vi "Nod eID handler.vi"(1 "Loop ID":T1, 11 "error in (no error)":errorcluster) -> ()   [LabVIEW 2011]
uses:
  Application Structure/Loop ID.ctl
  Defenitions/LEIN STAT 15 Id system cluster v2 wo lables.ctl
  emi Lib/System 01/0 - General/App/Loop control 2/Private/_emi_ SMLoop start condition.vi
  emi Lib/System 01/0 - General/App/Loop control 2/Private/_emi_ SMLoop Error Check.vi
  emi Lib/Basic/0 - General/Error/emi_Is Error.vi
  emi Lib/System 01/0 - General/App/Loop control 2/Private/_emi_SMLoop Register new.vi
  emi Lib/System 01/0 - General/S&E reporting/emi_Send S&E Error message.vi
  emi Lib/Basic/0 - General/Error/emi_ Is Error state.vi
  emi Lib/System 01/0 - General/emi_Read System ID.vi
  emi Lib/System 01/0 - General/App/Loop control/Private/_emi_GFV Loop Linking.vi
  emi Lib/System 01/0 - General/App/Loop control/Private/_emi_GFV Loop Enable.vi
  emi Lib/System 01/0 - General/App/Loop control 2/Private/_emi_ SMLoop Restart.vi
  emi Lib/System 01/0 - General/App/Private/_emi_GFV App Close.vi
  emi Lib/System 01/0 - General/App/Loop control 2/Private/_emi_ SMLoop Restart Counter.vi
  emi Lib/System 01/0 - General/App/Loop control/Private/_emi_GFV Loop Running.vi
  emi Lib/System 01/0 - General/Private/_emi_GFV System ID.vi
  emi Lib/System 01/0 - General/S&E reporting/Private/_emi_S&E Q Generator.vi
  <vilib>/Utility/error.llb/Clear Errors.vi
  emi Lib/System 01/0 - General/App/Loop control/Private/_emi_GFV stop a loop so it can reset.vi
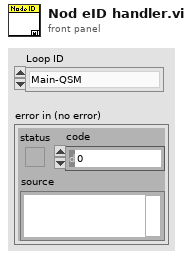
[diagram p1: front panel]
types:
  T1 = typedef "Loop ID.ctl" = enum16{"Main-QSM", "Main-Dialog", "Main-Ind Upd", "Main-Graph Upd", "Main-Debug", "Main-DebugW1", "Main-DebugW2", "Main-SE Handler", "Interface-PCP", "Interface-CANbus", "Interface-Modem", "Var Handling-Beat", "Var Handling-From PCP", "Var Handling-File storage", "Var Handling-From Simulator", "GUI-GrphW Mast", "GUI-GrphW Slav", "SIM-Tool W1", "SIM-Tool W2", "Alm-Sound", "LEIN-motor", "Tool data gatherer Qer", "Tool Data LEIN STAT2 dekoder", "Indicator Value Update", "Tool STAT2 dedicated reader", "Tool ID handler", "Detail View L1", "Detail View L2", "Main display enable view", "Sequence runner", "Voltage setpoint", "Resistance setpoint", "Stroker Wizard L1", "Stroker Wizard L2", "Alarm Handling", "Annotations Tip Strip", "Magna Interface", "Modem Status", "Var Handling - Modem Status", "Power interface detector"}
  T2 = typedef "LEIN STAT 15 Id system cluster v2 wo lables.ctl" = cluster{"LEIN version":u8, "LEIN implementation code":u8, "Serial number":u16, "Project":u16, "HW ID":u8, "FW ID":u8, "HW REV":u8, "FW REV":u8}
  T3 = enum16{"big-endian, network order", "native, host order", "little-endian"}
  T4 = typedef "_emi_ SMLoop sates.ctl" = enum16{"Init", "Standby", "Start", "Normal Operation", "Stop", "Error Handling", "End", "Post"}
  T5 = typedef "LEIN custom reply Q.ctl" = refnum<queue>
  T6 = typedef "LEIN Reply Holder.ctl" = cluster{"Reply msg(cmdif no reply)":T7, "Reply time":timestamp, "Valid reply":bool}
  T7 = typedef "LEIN CMD Cluster.ctl" = cluster{"SID":u8, "ANF":bool, "CMD":T8, "DATA":u8[]}
  T8 = typedef "LEIN CMD List.ctl" = enum8{"ACTI", "TASK", "RES0", "STAT", "RES1", "RES2", "RES3", "USER"}
  T9 = typedef "List of tools.ctl" = enum16{"Stroker", "Driller", "Tractor"}
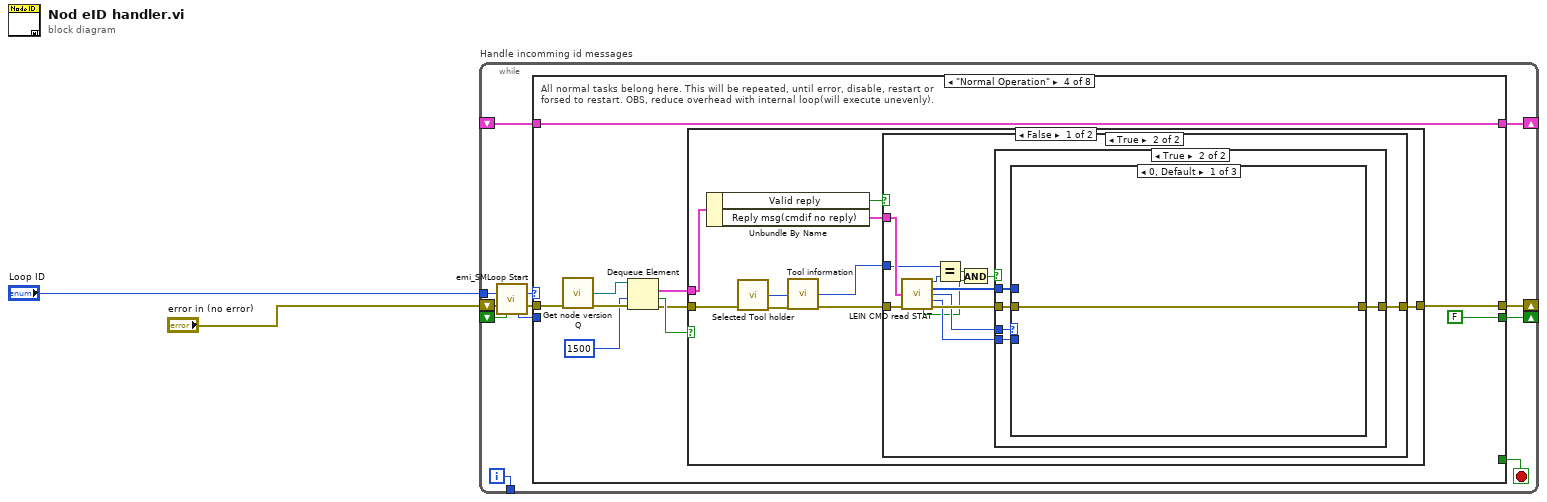
[diagram p0: block diagram]
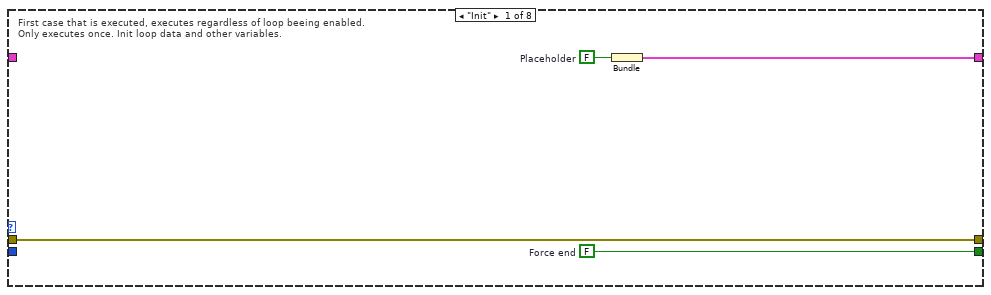
[diagram p2: hidden frame]
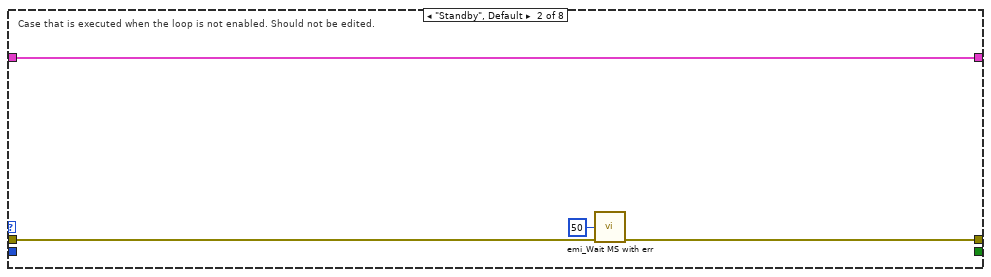
[diagram p3: hidden frame]
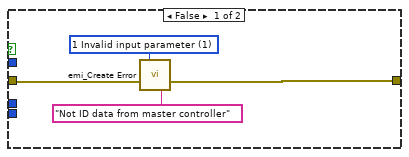
[diagram p6: hidden frame]
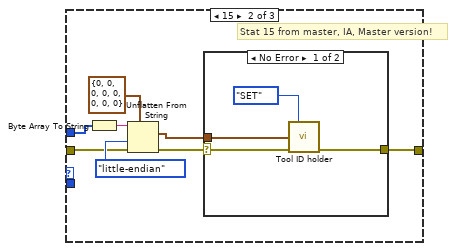
[diagram p7: hidden frame]
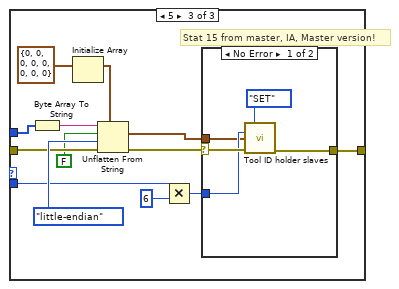
[diagram p9: hidden frame]
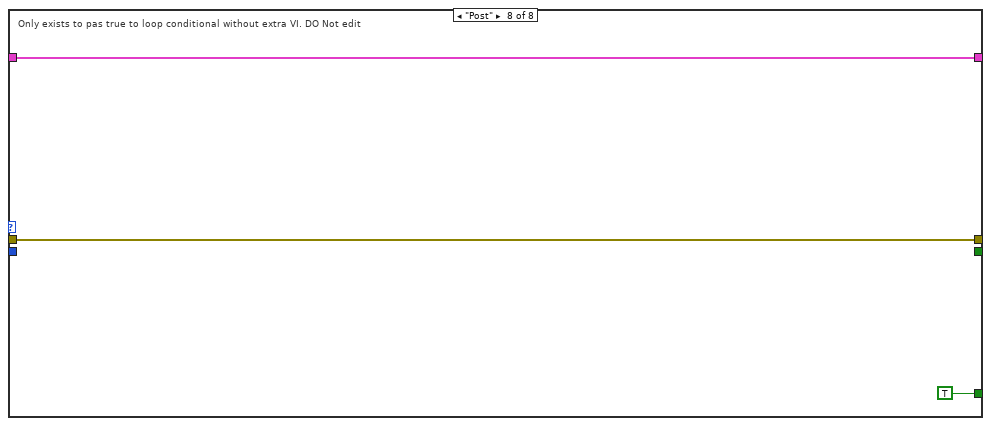
[diagram p15: hidden frame]
diagram:
  n1 = while "Handle incomming id messages" {
    shift-right: [w14] -> _
    shift-left: _ -> [w10]
    shift-right: [w12] -> _
    shift-left: "error in (no error)" -> [w8]
    tunnel: [w11] -> _
    shift-right: [w9] -> _
    shift-left: _ -> [w4]
    tunnel: "Loop ID" -> [w5]
    i -> [w11]
    stop <- w13 stop-if-true
    n2 = call "emi_SMLoop Start.vi"("Loop ID"=w5, "error in (no error)"=w8, "Force Stop(F)"=w4) -> ("Loop command"=w6:T4, "error out"=w7:errorcluster, "Loop ID out"=w3:i32)  [unwired: 10 in]
    n3 = case shown="\"Normal Operation\"" w6 {
      tunnel: [w17 w19 w23 w34 w100 w103 w104 w107] -> w14
      tunnel: [_ _ _ _ _ _ _ TRUE] -> w13
      tunnel: w7 -> [w18 w21 w24 w32 w101 w102 w105 w108]
      tunnel: [w18 w20 w24 w27 w101 w102 w105 w108] -> w12
      tunnel: w10 -> [_ w19 w23 w34 w100 w103 w104 w107]
      tunnel: [w15 _ _ FALSE ("Force End") _ _ _ _] -> w9
      tunnel: w3 -> [_ _ _ _ _ _ _ _]
      frame "Init" {
        w15 = FALSE  # Force end
        w16 = FALSE  # Placeholder
        # "First case that is executed, executes regardless of loop beeing enabled.\nOnly executes once. Init loop data and other variables."
        n4 = Bundle("Placeholder"=w16) -> (w17:cluster{"Placeholder":bool})  [unwired: 1 in]
      }
      frame "Standby", Default {
        # "Case that is executed when the loop is not enabled. Should not be edited."
        n5 = call "emi_Wait MS with err.vi"("milliseconds to wait(0)"=u32 50, "error in (no error)"=w21) -> ("error out"=w20:errorcluster)  [unwired: 13 in]
      }
      frame "Start" {
        # "Start or restart the loop. Should perform any init code. \nOpen channel and so on. Will perform each time the system is restarted."
      }
      frame "Normal Operation" {
        # "All normal tasks belong here. This will be repeated, until error, disable, restart or\nforsed to restart. OBS, reduce overhead with internal loop(will execute unevenly)."
        n6 = call "Get node version Q.vi"("error in"=w32) -> ("LEIN custom reply Q"=w30:T5, "error out"=w31:errorcluster)  [unwired: 13 in]
        n7 = Dequeue Element(queue=w30, timeout in ms (-1)=1500, error in (no error)=w31) -> (element=w25:T6, timed out?=w28:bool, error out=w26:errorcluster)  [unwired: 1 out]
        n8 = case shown="False" w28 {
          tunnel: [w41 w99] -> w27
          tunnel: w26 -> [w37 w99]
          tunnel: w25 -> [w43 _]
          frame False {
            n9 = Unbundle By Name(w43) -> ("Valid reply"=w42:bool, "Reply msg(cmdif no reply)"=w40:T7)
            n10 = call "Selected Tool holder.vi"("error in (no error)"=w37) -> ("Tool out"=w39:T9, "error out"=w38:errorcluster)  [unwired: 13 in]
            n11 = call "Tool information.vi"("Tool in"=w39, "error in (no error)"=w38) -> ("Main node address"=w35:u8, "error out"=w36:errorcluster)  [unwired: 10 in, 2 out]
            n12 = case shown="True" w42 {
              tunnel: w36 -> [w44 w55]
              tunnel: [w44 w56] -> w41
              tunnel: w40 -> [_ w54]
              tunnel: w35 -> [_ w45]
              frame False {
              }
              frame True {
                n13 = call "LEIN CMD read STAT.vi"("CMD"=w54, "error in (no error)"=w55) -> ("SID"=w49:u8, "Data"=w53:u8[], "STAT ID"=w51:u8, "STAT Part"=w50:u8, "ACK"=w46:bool, "error out"=w52:errorcluster)  [unwired: 8 in]
                n14 = Equal?(x=w45, y=w49) -> (x = y?=w47:bool)
                n15 = And(x=w47, y=w46) -> (x .and. y?=w48:bool)
                n16 = case shown="True" w48 {
                  tunnel: w52 -> [w60 w64]
                  tunnel: [w59 w65] -> w56
                  tunnel: w51 -> [_ w63]
                  tunnel: w53 -> [_ w62]
                  tunnel: w50 -> [_ w61]
                  frame False {
                    w58 = 1 items=["0 No Error"=0, "1 Invalid input parameter"=1, "6 Generic file IO "=6, "7 File not Found"=7, "35 Generic Pring Error"=35, "37 Device not Found"=37, "39 Device Unit Error"=39, "40 Could fot Open Device"=40, "42 Generic Error"=42, "52 Unknown Message"=52, "98 Bad File type"=98, "99 Bad File Version"=99, "100 Bad Data in File"=100, "1018 Unspecefied Error"=1018, "1041 Incorrect Password"=1041, "1043 Feature not in this version"=1043, "1109 Unsuported Data type"=1109, "1444 Did not close sucessfully"=1444] ("Error Code")
                    n17 = call "emi_Create Error.vi"("Error Code"=w58, "error in (no error)"=w60, "Append String(\"\")"="Not ID data from master controller" ("Append String(\"\")")) -> ("error out"=w59:errorcluster)  [unwired: 12 in]
                  }
                  frame True {
                    n18 = case shown="0, Default" w63 {
                      tunnel: [w66 w69 w82] -> w65
                      tunnel: w64 -> [w66 w72 w90]
                      tunnel: w62 -> [_ w71 w89]
                      tunnel: w61 -> [_ _ w85]
                      frame 0, Default {
                      }
                      frame 15 {
                        # "Stat 15 from master, IA, Master version!"
                        n19 = Byte Array To String(unsigned byte array=w71) -> (string=w73:string)
                        n20 = Unflatten From String(type=T2 {"LEIN version"=0, "LEIN implementation code"=0, "Serial number"=0, "Project"=0, "HW ID"=0, "FW ID"=0, "HW REV"=0, "FW REV"=0} ("Solenoid"), binary string=w73, byte order (0:big-endian, network order)=T3."little-endian", error in (no error)=w72) -> (value=w68:T2, error out=w67:errorcluster)  [unwired: 1 in, 1 out]
                        n21 = case shown="No Error" w67 {
                          selector: w67 -> [w75 w79]
                          tunnel: [w78 w79] -> w69
                          tunnel: w68 -> [w77 _]
                          frame No Error {
                            n22 = call "Tool ID holder.vi"("Action(GET)"=enum16{"GET", "SET"}."SET", "value in"=w77, "error in (no error)"=w75) -> ("error out"=w78:errorcluster)  [unwired: 11 in, 1 out]
                          }
                          frame Error {
                          }
                        }
                      }
                      frame 5 {
                        # "Stat 15 from master, IA, Master version!"
                        n23 = Byte Array To String(unsigned byte array=w89) -> (string=w91:string)
                        n24 = Initialize Array(T2 {"LEIN version"=0, "LEIN implementation code"=0, "Serial number"=0, "Project"=0, "HW ID"=0, "FW ID"=0, "HW REV"=0, "FW REV"=0} ("Solenoid")) -> (w86:T2[])  [unwired: 1 in]
                        n25 = Unflatten From String(type=w86, binary string=w91, data includes array or string size? (T)=FALSE, byte order (0:big-endian, network order)=T3."little-endian", error in (no error)=w90) -> (value=w80:T2[], error out=w83:errorcluster)  [unwired: 1 out]
                        n26 = Multiply(x=w85, y=u8 6) -> (x*y=w81:u8)
                        n27 = case shown="No Error" w83 {
                          selector: w83 -> [w97 w98]
                          tunnel: [w96 w98] -> w82
                          tunnel: w81 -> [w95 _]
                          tunnel: w80 -> [w94 _]
                          frame No Error {
                            n28 = call "Tool ID holder slaves.vi"("Action(GET)"=enum16{"GET", "SET"}."SET", "Set index"=w95, "value in"=w94, "error in (no error)"=w97) -> ("error out"=w96:errorcluster)  [unwired: 10 in, 1 out]
                          }
                          frame Error {
                          }
                        }
                      }
                    }
                  }
                }
              }
            }
          }
          frame True {
          }
        }
      }
      frame "Stop" {
        # "Stop the loop. May be restarted later. Close interfaces and the like"
      }
      frame "Error Handling" {
        # "Loop automaticaly returns here after error is found. If error is cleared, \nLoop wil continue as normal(if was operative when error."
      }
      frame "End" {
        # "Only executes at application end has. Should performa any action the loop \nneeds to finnish. Executes only once."
      }
      frame "Post" {
        # "Only exists to pas true to loop conditional without extra VI. DO Not edit"
      }
    }
  }
